vi "rejestr_PH.vi"() -> ()   [LabVIEW 2021]
panel:
  out "Wynik":dbl
  in  "Numer obliczanego wyrazu":dbl
  in  "Ró¿nica":dbl
  in  "Pierwszy wyraz":dbl
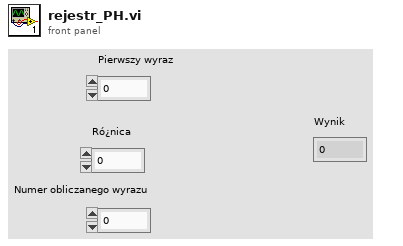
[diagram p1: front panel]
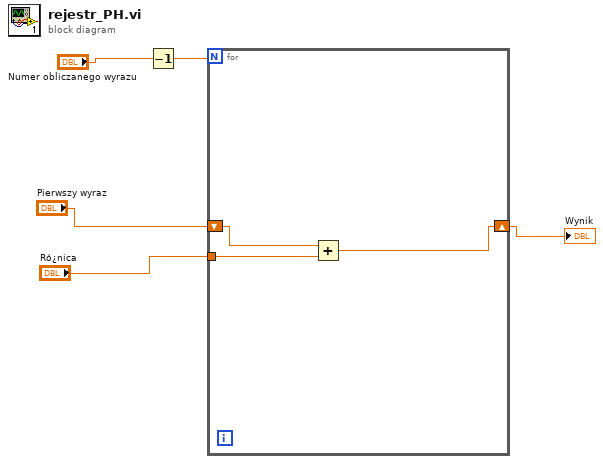
[diagram p0: block diagram]
diagram:
  n1 = Decrement(x="Numer obliczanego wyrazu") -> (x-1=w4:dbl)
  n2 = for {
    N: w4 -> [_]
    shift-right: [w6] -> w1
    shift-left: "Pierwszy wyraz" -> [w7]
    tunnel: "Ró¿nica" -> [w8]
    n3 = Add(x=w7, y=w8) -> (x+y=w6:dbl)
  }
  "Wynik" <- w1
